vi "POST Template.vi"(8 "error in":errorcluster, 11 "Nominal Client in":refnum<class "Nominal Client.lvclass">) -> (0 "error out":errorcluster, 2 "Response":string, 3 "Nominal Client out":refnum<class "Nominal Client.lvclass">)   [LabVIEW 2020]
doc: "This template lets end users extend the Nominal LabVIEW Client without waiting for Nominal to implement new functionality.\n\nDropping this template onto your block diagram drops the code directly, not a subVI.\n\nSave VIs created from this template in your project source code, not the toolkit source code, as they will be removed when the toolkit updates.\n\nIf you would like to contribute to the Nominal LabVIEW Client toolkit, speak to a member of our team."
uses:
  Nominal Client/Nominal Client.lvclass/Nominal Client.ctl
  Nominal Client/create.authorization_header.vi
  Nominal Client/trace.payload_sent.vi
  Nominal Client/trace.payload_received.vi
  Nominal Client/error.vi
  Nominal Client/api_token.get.vi
  Nominal Client/trace.calling_method.vi
  <vilib>/JDP Science/JDP Science Common Utilities/Trim Whitespace__JDP.vi
  <vilib>/AdvancedString/1D String Array to Delimited String.vi
  Nominal Client/error.vi/859f8e04-e495-489b-b5b4-7ac163f56130.vi
  <vilib>/Utility/libraryn.llb/Get File Extension.vi
  Nominal Client/log_file.write.vi
  submodules/reqwest-labview/lv-src/reqwest/get.vi
  <vilib>/JDP Science/JSONtext/Get all Object Items.vi
  <vilib>/Utility/error.llb/Error Cluster From Error Code.vi
  <vilib>/JDP Science/JSONtext/JSON text to Variant.vi
  <vilib>/JDP Science/JSONtext/LVClass Serializer/JSONtext LVClass Serializer.lvclass
  Nominal Client/Nominal Client.lvclass
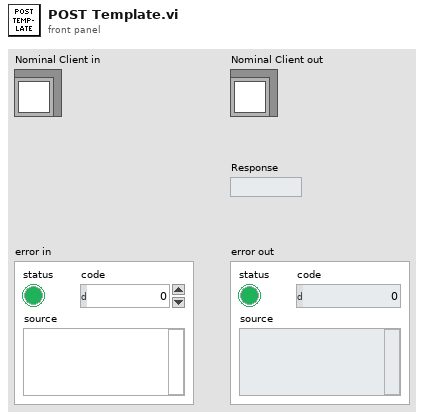
[diagram p1: front panel]
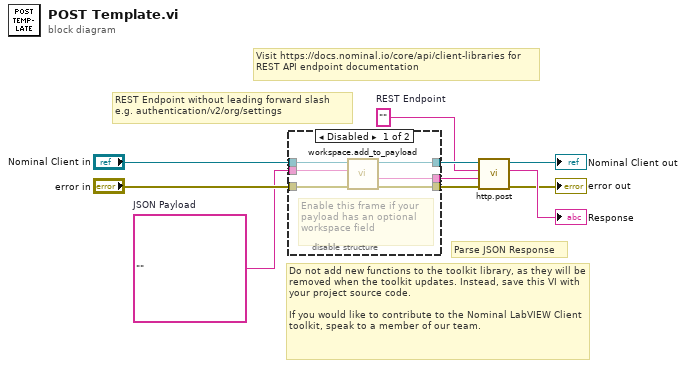
[diagram p0: block diagram]
diagram:
  w2 = ""  # JSON Payload
  w8 = ""  # REST Endpoint
  # "Do not add new functions to the toolkit library, as they will be removed when the toolkit updates. Instead, save this VI with your project source code.\n\nIf you would like to contribute to the Nominal LabVIEW Client toolkit, speak to a member of our team."
  # "Parse JSON Response"
  # "REST Endpoint without leading forward slash\ne.g. authentication/v2/org/settings"
  # "Visit https://docs.nominal.io/core/api/client-libraries for REST API endpoint documentation"
  n1 = disable-structure shown="Disabled" {
    disable-tunnel: [w16 w19] -> w10
    disable-tunnel: [w15 w17] -> w9
    disable-tunnel: "Nominal Client in" -> [w14 w19]
    disable-tunnel: "error in" -> [w13 w18]
    disable-tunnel: [w12 w18] -> w3
    disable-tunnel: w2 -> [w11 w17]
    frame Disabled {
      # "Enable this frame if your payload has an optional workspace field"
      n2 = call "workspace.add_to_payload.vi"("error in"=w13, "JSON payload in"=w11, "Nominal Client in"=w14) -> ("error out"=w12:errorcluster, "JSON payload out"=w15:string, "Nominal Client out"=w16:refnum<class "Nominal Client.lvclass">)  [unwired: 6 in]
    }
    frame Enabled {
    }
  }
  n3 = call "http.post.vi"("error in"=w3, "Request body"=w9, "Path"=w8, "Nominal Client in"=w10) -> ("error out"=→"error out":errorcluster, "Response"=→"Response":string, "Nominal Client out"=→"Nominal Client out":refnum<class "Nominal Client.lvclass">)  [unwired: 5 in]
